vi "yakup_demiryurek18.vi"() -> ()   [LabVIEW 2020]
uses:
  <vilib>/express/express analysis/Spectral/Block/exnSpectralBlock spectral measurements PSD poly.vi
  <vilib>/express/express analysis/Spectral/Block/exnSpectralBlock spectral measurements PSD DDT.vi
  <vilib>/express/express analysis/Spectral/XNode/ExpressSpectralMeasurementsBlockNode.xnode
panel:
  out "Original Signal 4":dynamicdata(graph) caption="Sine"
  out "Genlik Modülasyonu":dynamicdata(graph) caption="Sine"
  out "Taşıyıcı":dynamicdata(graph) caption="Sine"
  in  "Am":dbl
  in  "Fm":dbl
  out "Mu":dbl
  out "Mesaj":dynamicdata(graph) caption="Sine"
  in  "Ac":dbl
  in  "Fc":dbl
  in  "Ka":dbl
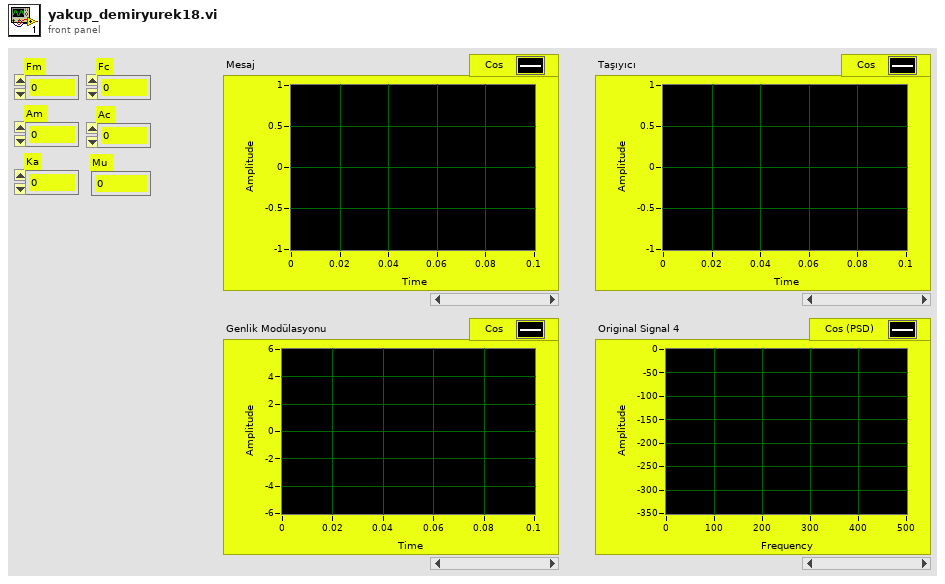
[diagram p1: front panel]
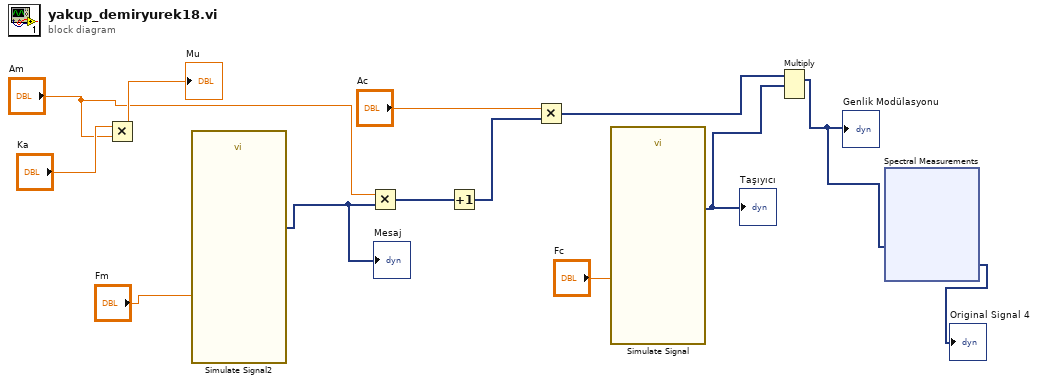
[diagram p0: block diagram]
diagram:
  n1 = Multiply(x="Ka", y="Am") -> (x*y=→"Mu":dbl)
  n2 = call "Simulate Signal2"("Frequency"="Fm") -> ("Cos"=w8:dynamicdata)  [unwired: 13 in, 1 out]
  "Mesaj" <- w8
  n3 = Multiply(x="Am", y=w8) -> (x*y=w11:dynamicdata)
  n4 = Increment(x=w11) -> (x+1=w13:dynamicdata)
  n5 = Multiply(x="Ac", y=w13) -> (x*y=w7:dynamicdata)
  n6 = call "Simulate Signal"("Frequency"="Fc") -> ("Cos"=w6:dynamicdata)  [unwired: 13 in, 1 out]
  "Taşıyıcı" <- w6
  n7 = Multiply(1:w6, 2:w7) -> (0:w2:dynamicdata)  [unwired: 1 in, 1 out]
  "Genlik Modülasyonu" <- w2
  n8 = xnode "Spectral Measurements"("Signals"=w2) -> ("PSD"=→"Original Signal 4":dynamicdata)  [unwired: 1 in, 1 out]
